vi "sArduinoParse.vi"(0 "read buffer":string, 1 "Expected Arduino Parameters":i32=8) -> (2 "Number Arduino Parameters":i32, 3 "Arduino Data Names":string[](array[string]), 4 "Arduino Data":dbl[](array[numeric]), 5 "Data good?":bool)   [LabVIEW 2014]
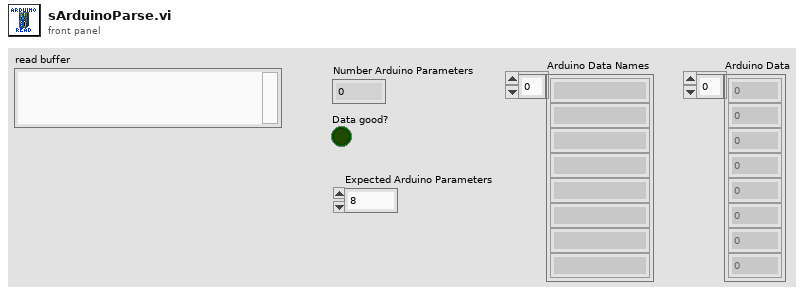
[diagram p1: front panel]
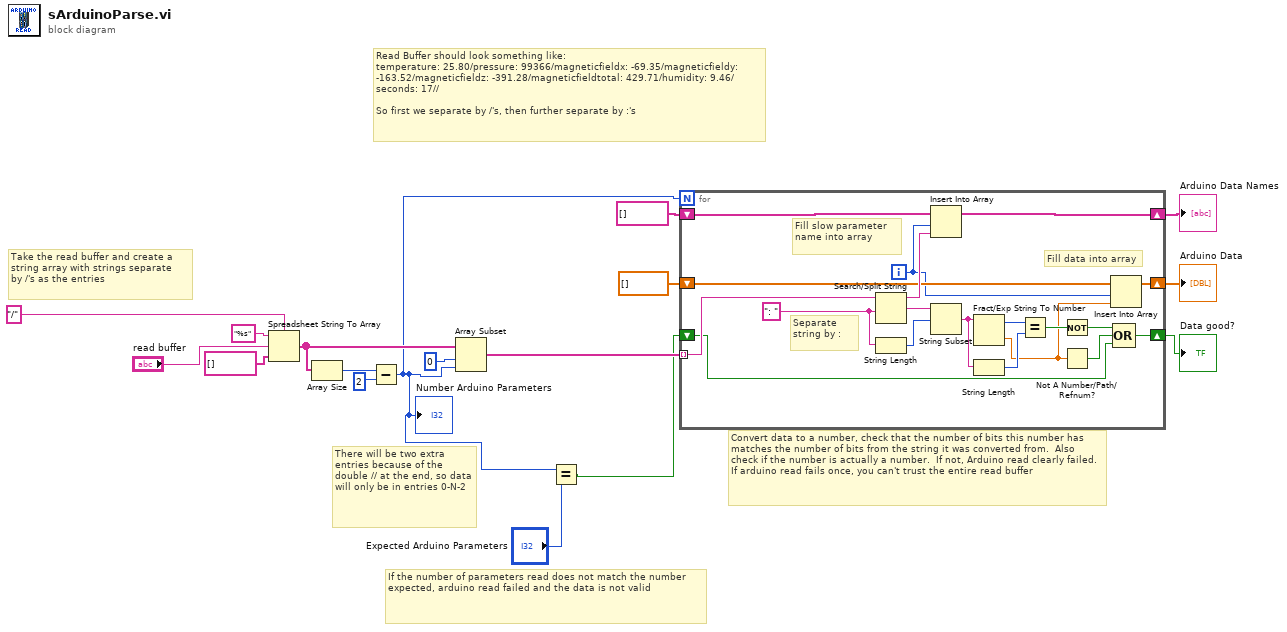
[diagram p0: block diagram]
diagram:
  # "If the number of parameters read does not match the number expected, arduino read failed and the data is not valid"
  # "Convert data to a number, check that the number of bits this number has matches the number of bits from the string it was converted from.  Also check if the number is actually a number.  If not, Arduino read clearly failed.  If arduino read fails once, you can't trust the entire read buffer"
  # "Read Buffer should look something like:\ntemperature: 25.80/pressure: 99366/magneticfieldx: -69.35/magneticfieldy: -163.52/magneticfieldz: -391.28/magneticfieldtotal: 429.71/humidity: 9.46/seconds: 17//\n\nSo first we separate by /'s, then further separate by :'s"
  # "There will be two extra entries because of the double // at the end, so data will only be in entries 0-N-2"
  # "Take the read buffer and create a string array with strings separate by /'s as the entries"
  n1 = Spreadsheet String To Array(delimiter (Tab)="/", format string="%s", spreadsheet string="read buffer", array type (2D Dbl)=string[] []) -> (array=w12:string[])
  n2 = Array Size(array=w12) -> (size(s)=w11:i32)
  n3 = Subtract(x=w11, y=2) -> (x-y=w3:i32)
  "Number Arduino Parameters" <- w3
  n4 = Array Subset(array=w12, index=0, length=w3) -> (w7:string[])
  n5 = Equal?(x=w3, y="Expected Arduino Parameters") -> (x = y?=w1:bool)
  n6 = for {
    N: w3 -> [_]
    shift-right: [w28] -> w6
    shift-left: string[] [] ("array type (2D Dbl)") -> [w30]
    shift-right: [w20] -> w4
    shift-left: dbl[] [] ("array type (2D Dbl)") -> [w23]
    tunnel: w7 -> [w31] mode=indexing
    shift-right: [w25] -> w5
    shift-left: w1 -> [w24]
    i -> [w22]
    w19 = ": " ("search string/char (-)")
    # "Fill data into array"
    # "Fill slow parameter name into array"
    # "Separate string by :"
    n7 = Search/Split String(string=w31, search string/char (-)=w19) -> (substring before match=w29:string, match + rest of string=w32:string)  [unwired: 1 in, 1 out]
    n8 = String Length(string=w19) -> (length=w18:i32)
    n9 = Insert Into Array(array=w30, index=w22, new element=w29) -> (w28:string[])
    n10 = String Subset(string=w32, offset (0)=w18) -> (substring=w33:string)  [unwired: 1 in]
    n11 = Fract/Exp String To Number(string=w33) -> (offset past number=w36:i32, number=w21:dbl)  [unwired: 3 in]
    n12 = String Length(string=w33) -> (length=w35:i32)
    n13 = Equal?(x=w36, y=w35) -> (x = y?=w34:bool)
    n14 = Not(x=w34) -> (.not. x?=w27:bool)
    n15 = Not A Number/Path/Refnum?(number/path/refnum=w21) -> (NaN/Path/Refnum?=w26:bool)
    n16 = Insert Into Array(array=w23, index=w22, new element=w21) -> (w20:dbl[])
    n17 = Compound Arithmetic op=OR(w27, w26, w24) -> (w25:bool)
  }
  "Arduino Data Names" <- w6
  "Data good?" <- w5
  "Arduino Data" <- w4
